vi "Dither.vi"(0 "Moisture (V) in":dbl=2.5, 5 "Dither":dbl=0.05, 7 "Iteration Terminal":i32, 11 "Error In":errorcluster) -> (8 "Moisture (V)":dbl, 15 "Error Out":errorcluster)   [LabVIEW 2021]
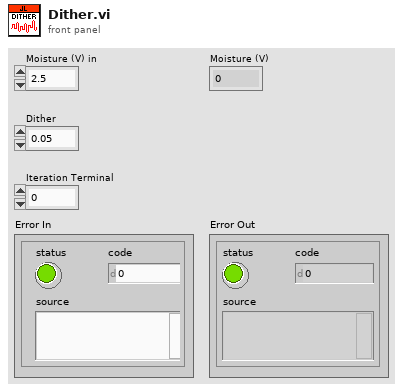
[diagram p1: front panel]
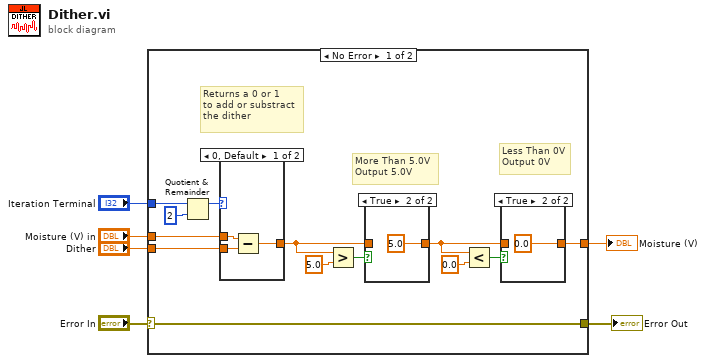
[diagram p0: block diagram]
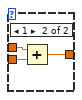
[diagram p4: hidden frame]
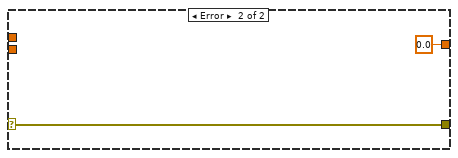
[diagram p5: hidden frame]
diagram:
  n1 = case shown="No Error" "Error In" {
    selector: "Error In" -> [w7 w31]
    tunnel: [w18 0.0 ("y")] -> w6
    tunnel: "Iteration Terminal" -> [w11 _]
    tunnel: "Dither" -> [w10 _]
    tunnel: "Moisture (V) in" -> [w8 _]
    tunnel: [w7 w31] -> w1
    frame No Error {
      # "Returns a 0 or 1\nto add or substract\nthe dither"
      # "More Than 5.0V\nOutput 5.0V"
      # "Less Than 0V\nOutput 0V"
      n2 = Quotient & Remainder(x=w11, y=2) -> (x-y*floor(x/y)=w9:i32)  [unwired: 1 out]
      n3 = case shown="0, Default" w9 {
        tunnel: [w26 w29] -> w19
        tunnel: w8 -> [w25 w28]
        tunnel: w10 -> [w24 w27]
        frame 0, Default {
          n4 = Subtract(x=w25, y=w24) -> (x-y=w26:dbl)
        }
        frame 1 {
          n5 = Add(x=w28, y=w27) -> (x+y=w29:dbl)
        }
      }
      n6 = Greater?(x=w19, y=5.0) -> (0:w15:bool)
      n7 = case shown="True" w15 {
        tunnel: [w22 5.0 ("y")] -> w17
        tunnel: w19 -> [w22 _]
        frame False {
        }
        frame True {
        }
      }
      n8 = Less?(x=w17, y=0.0) -> (x < y?=w13:bool)
      n9 = case shown="True" w13 {
        tunnel: [w20 0.0 ("y")] -> w18
        tunnel: w17 -> [w20 _]
        frame False {
        }
        frame True {
        }
      }
    }
    frame Error {
    }
  }
  "Moisture (V)" <- w6
  "Error Out" <- w1
